vi "Main.vi"(8 "error in":errorcluster, 11 "Camera detection in":refnum<class "Camera detection.lvclass">) -> (0 "error out":errorcluster, 3 "Camera detection out":refnum<class "Camera detection.lvclass">)   [LabVIEW 2026, in "Camera detection.lvclass"]
doc: "The <b>Queued Message Handler</b> of the Worker that owns this VI."
uses:
  Camera detection.lvclass
  C:/Program Files/National Instruments/LabVIEW 2026/vi.lib/addons/_Workers/Library/Classes/Worker/Worker.lvclass
  Initialization Data.ctl
  Response Cases.ctl
  Camera detection.lvclass/Camera detection.ctl
  rql_Open Camera.ctl
  81cbe082-1300-4c77-b04d-38d83d7810f2.vi
  <vilib>/Utility/error.llb/Error Cluster From Error Code.vi
  <vilib>/ErrorRing/Error Ring.xnode
  <vilib>/addons/_Workers/Library/Classes/Message Queue/Message Queue.lvclass
  <vilib>/addons/_Workers/Debugger/Debug Client/Debug Client.lvlib
  <vilib>/Serenial/G Industrial Camera/g_industrial_cam/g_industrial_cam.lvlib
panel:
  out "élément":string
  in  "Open":bool
  in  "Caméra Identifiée":u16(ring) items=["Basler-acA640-120gm-22026460", "Basler-acA640-121gm-40611192"]
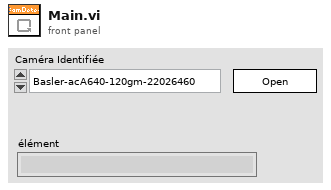
[diagram p1: front panel]
types:
  T1 = typedef "Camera detection.lvclass/Initialization Data.ctl" = cluster{"Response Cases":T2}
  T2 = typedef "Camera detection.lvclass/Response Cases.ctl" = cluster{"Placeholder - Can be deleted":string, "Non du VI":string, "Refnum Caméra ID":refnum<vi>}
  T3 = typedef "Camera detection.lvclass/rql_Open Camera.ctl" = cluster{"String":string, "Incr":i32}
  T4 = typedef "g_industrial_cam.lvlib/Device Enumeration.ctl" = cluster{"ID":string, "Protocol":string, "Vendor":string, "Model":string, "Serial":string, "Address":string}
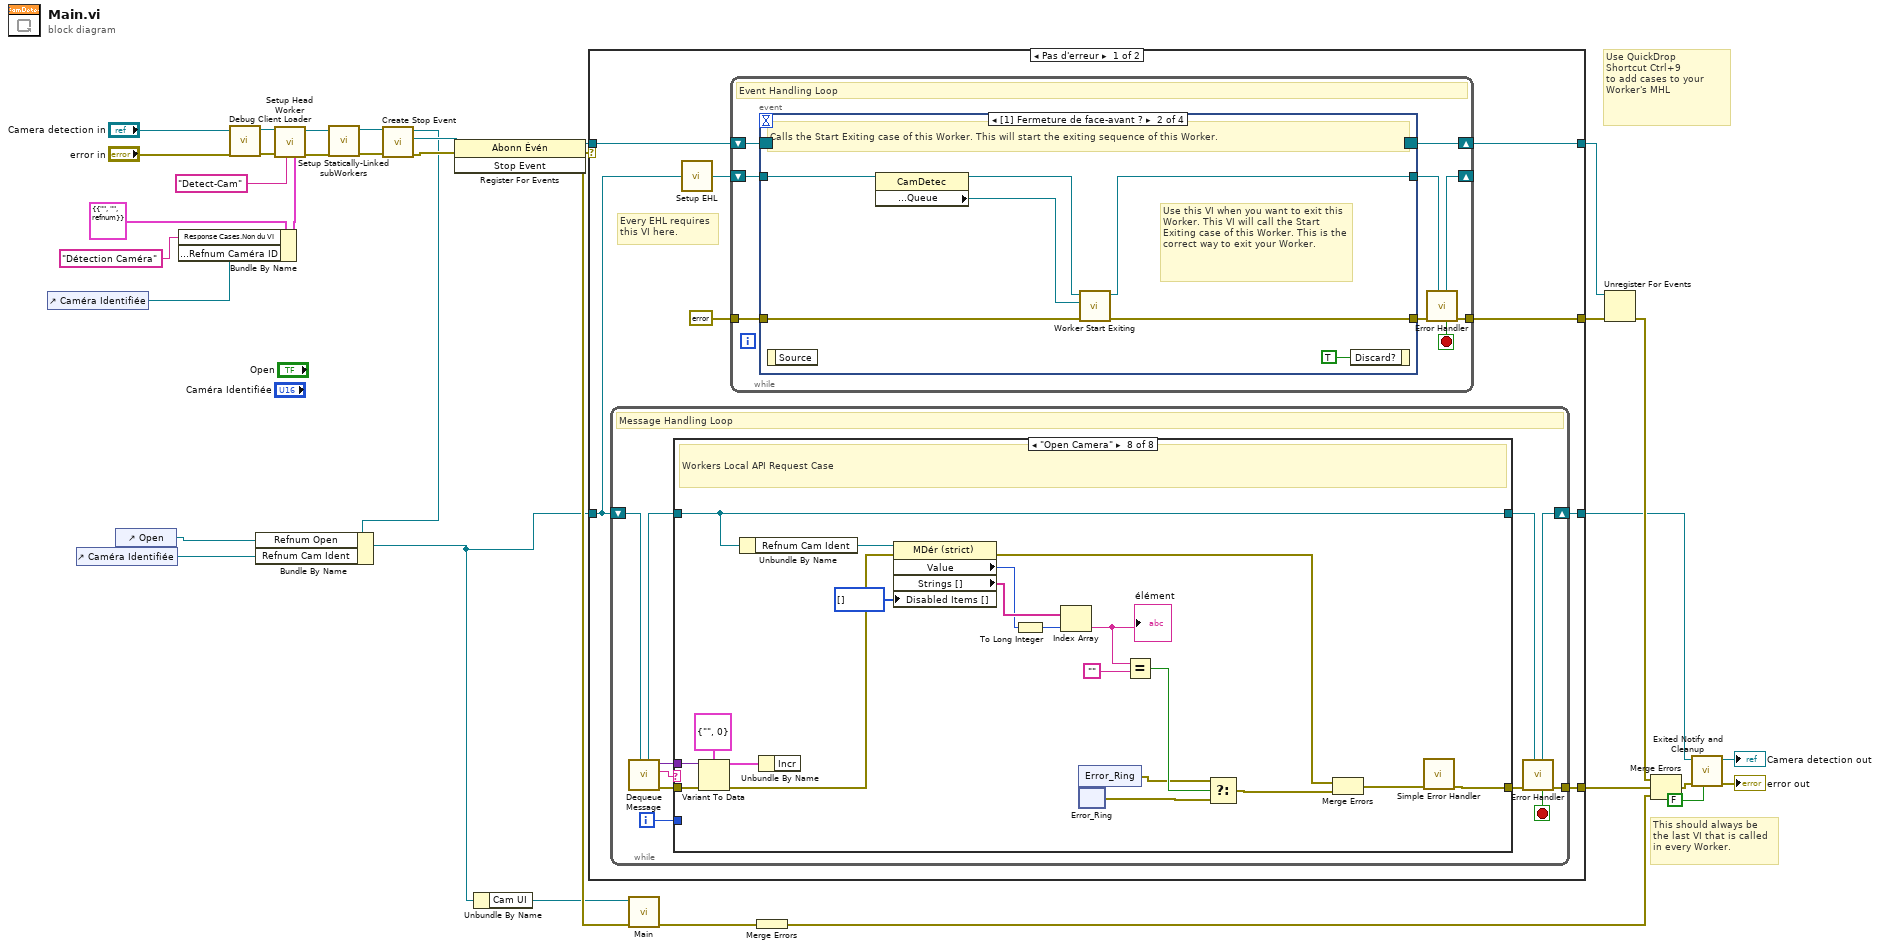
[diagram p0: block diagram]
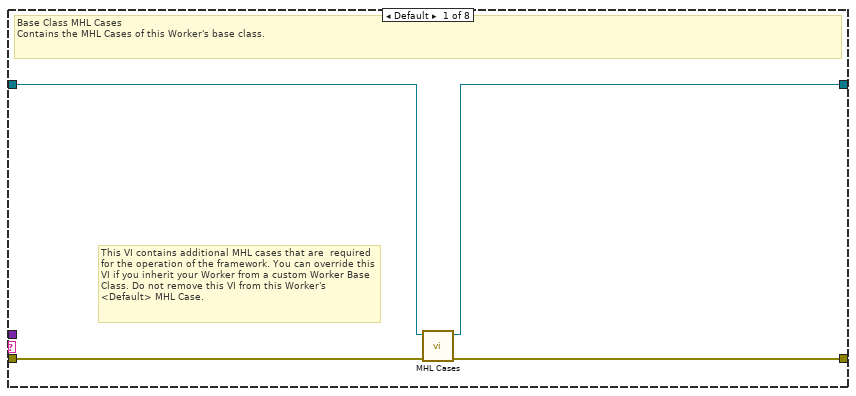
[diagram p2: hidden frame]
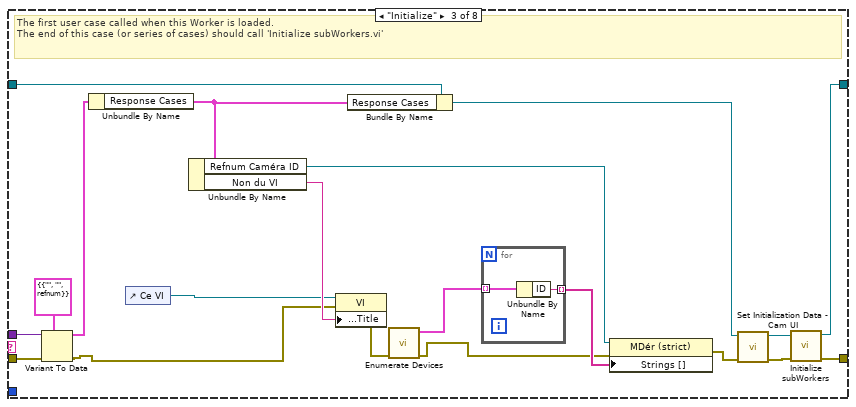
[diagram p4: hidden frame]
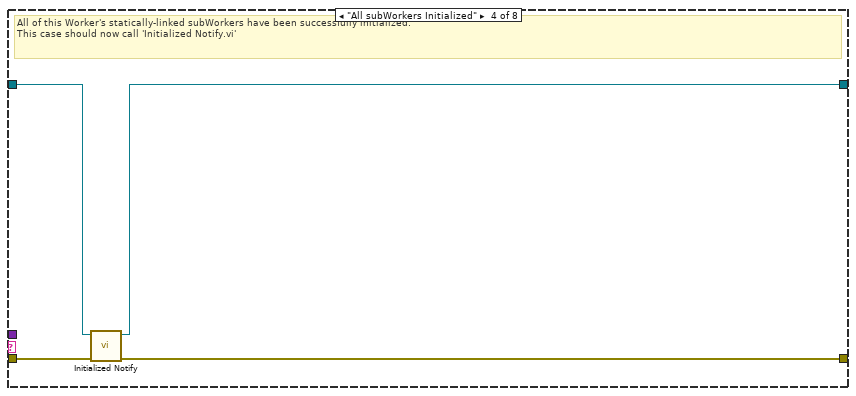
[diagram p5: hidden frame]
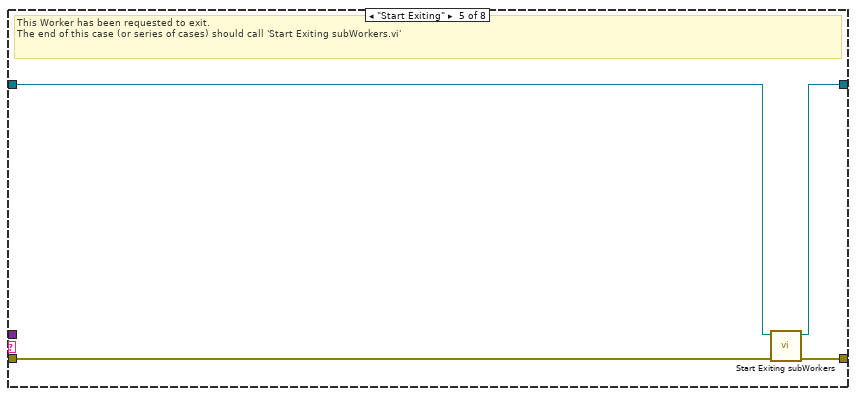
[diagram p6: hidden frame]
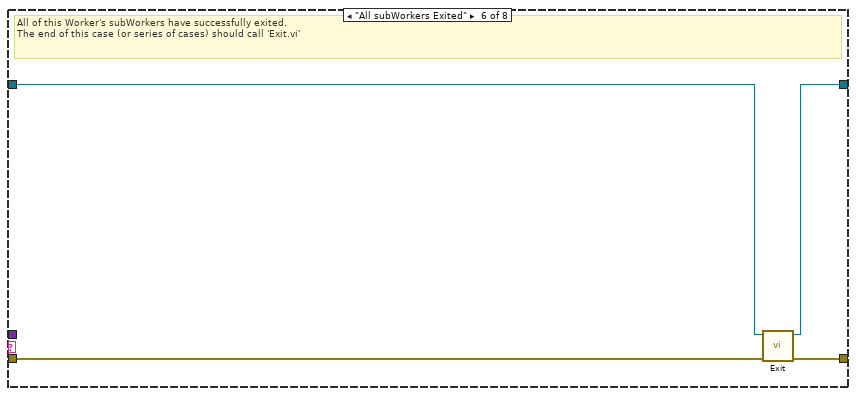
[diagram p7: hidden frame]
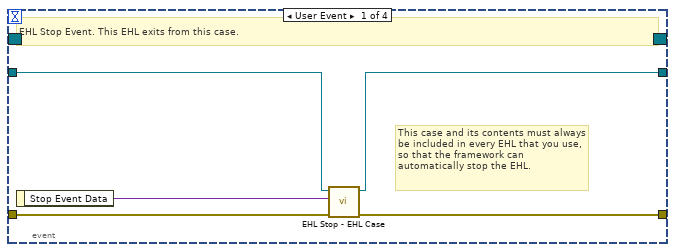
[diagram p9: hidden frame]
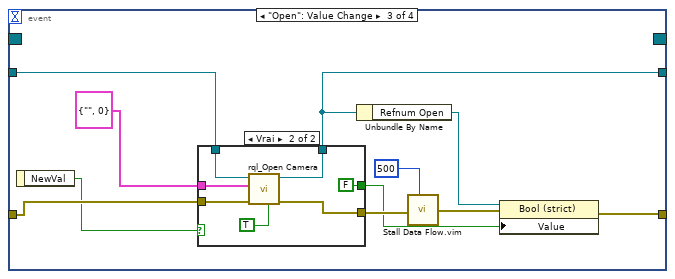
[diagram p10: hidden frame]
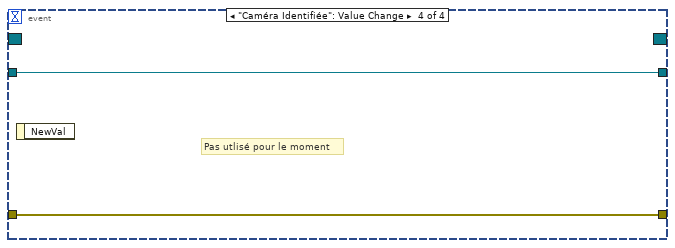
[diagram p12: hidden frame]
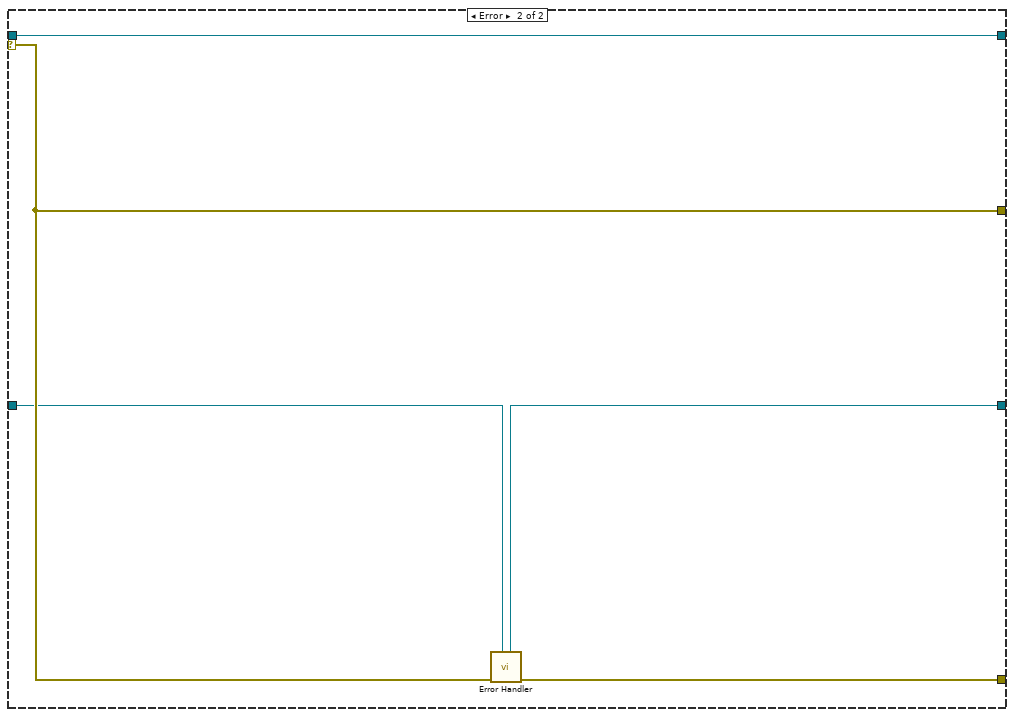
[diagram p13: hidden frame]
diagram:
  # "Use QuickDrop\nShortcut Ctrl+9\nto add cases to your\nWorker's MHL"
  # "This should always be the last VI that is called in every Worker."
  n1 = control-ref of="Caméra Identifiée"() -> (w13:refnum<vi>)
  n2 = control-ref of="Caméra Identifiée"() -> (w10:refnum<vi>)
  n3 = control-ref of="Open"() -> (w11:refnum<vi>)
  n4 = Bundle By Name ("Assembler par nom")(cluster=T1 {"Response Cases"={"Placeholder - Can be deleted"="", "Non du VI"="", "Refnum Caméra ID"=refnum}} ("Initialization Data"), "Response Cases.Non du VI"="Détection Caméra", "Response Cases.Refnum Caméra ID"=w13) -> (w16:T1)
  n5 = call <vilib>:"Debug Client Loader.vi"("error in (no error)"="error in", "Worker_"="Camera detection in") -> ("error out"=w19:errorcluster, "Worker_out"=w20:refnum<class "Camera detection.lvclass">)  [unwired: 8 in]
  n6 = call-dynamic "Setup Head Worker.vi"("Initalization Data"=w16, "Worker Alias"="Detect-Cam", "error in"=w19, "Worker_"=w20) -> ("error out"=w4:errorcluster, "Worker_out"=w3:refnum<class "Camera detection.lvclass">)  [unwired: 6 in]
  n7 = call "Setup Statically-Linked subWorkers.vi"("error in"=w4, "Camera detection in"=w3) -> ("error out"=w1:errorcluster, "Camera detection out"=w2:refnum<class "Camera detection.lvclass">)  [unwired: 8 in]
  n8 = call-dynamic "Create Stop Event.vi"("error in"=w1, "Worker"=w2) -> ("error out"=w28:errorcluster, "Stop Event"=w25:refnum<user-event>, "Worker out"=w22:refnum<class "Camera detection.lvclass">)  [unwired: 7 in]
  n9 = Bundle By Name ("Assembler par nom")(cluster=w22, "Refnum Open"=w11, "Refnum Cam Ident"=w10) -> (w12:refnum<class "Camera detection.lvclass">)
  n10 = register-events(error in=w28, w25) -> (reference out=w27:refnum<event-registration>, error out=w21:errorcluster)  [unwired: 1 in]
  n11 = Unbundle By Name(w12) -> ("Cam UI"=w7:refnum<class "Caméra UI.lvclass">)
  n12 = case shown="Pas d'erreur" w21 {
    tunnel: w12 -> [w36 w165]
    tunnel: [w34 w166] -> w26
    tunnel: w27 -> [w41 w167]
    tunnel: [w38 w168] -> w32
    tunnel: [w40 w167] -> w31
    tunnel: [w35 w164] -> w29
    selector: w21 -> [_ w168]
    frame No Error {
      # "Every EHL requires\nthis VI here."
      n13 = while {
        shift-right: [w50] -> w35
        shift-left: w36 -> [w52]
        tunnel: [w51] -> w34
        i -> [w43]
        stop <- w44 stop-if-true
        # "Message Handling Loop"
        n14 = call-dynamic "Dequeue Message.vi"("Worker"=w52) -> ("error out"=w49:errorcluster, "Case out"=w45:string, "Data out"=w42:variant, "Worker out"=w47:refnum<class "Camera detection.lvclass">)  [unwired: 6 in, 1 out]
        n15 = case "Worker MHL Case Structure (DO NOT CHANGE LABEL NAME)" shown="\"Open Camera\"" w45 {
          tunnel: w49 -> [w56 w57 w76 w82 w85 w92 w94 w114]
          tunnel: [w55 w57 w78 w81 w88 w91 w94 w98] -> w48
          tunnel: w47 -> [w54 w58 w75 w84 w86 w90 w93 w110]
          tunnel: [w53 w58 w77 w83 w87 w89 w93 w110] -> w46
          tunnel: w43 -> [_ _ _ _ _ _ _ _]
          tunnel: w42 -> [_ _ w74 _ _ _ _ w112]
          frame Default {
            # "This VI contains additional MHL cases that are  required for the operation of the framework. You can override this VI if you inherit your Worker from a custom Worker Base Class. Do not remove this VI from this Worker's <Default> MHL Case."
            # "Base Class MHL Cases\nContains the MHL Cases of this Worker's base class."
            n16 = call-dynamic "MHL Cases.vi"("error in"=w56, "Worker in"=w54) -> ("error out"=w55:errorcluster, "Worker out"=w53:refnum<class "Camera detection.lvclass">)  [unwired: 8 in]
          }
          frame "------------ FRAMEWORK CASES -----------" {
            # "Start of Workers Framework Cases"
          }
          frame "Initialize" {
            # "The first user case called when this Worker is loaded.\nThe end of this case (or series of cases) should call 'Initialize subWorkers.vi'"
            n17 = Variant To Data(error in=w76, type=T1 {"Response Cases"={"Placeholder - Can be deleted"="", "Non du VI"="", "Refnum Caméra ID"=refnum}} ("Initialization Data"), Variant=w74) -> (data=w73:T1, error out=w67:errorcluster)
            n18 = Unbundle By Name(w73) -> ("Response Cases"=w68:T2)
            n19 = control-ref of="Ce VI"() -> (w63:refnum<vi>)
            n20 = Unbundle By Name(w68) -> ("Refnum Caméra ID"=w65:refnum<vi>, "Non du VI"=w71:string)
            n21 = property class="VI"(reference=w63, error in=w67, "Front Panel.Title"=w71) -> (error out=w70:errorcluster)  [unwired: 1 out]
            n22 = Bundle By Name ("Assembler par nom")(cluster=w75, "Response Cases"=w68) -> (w59:refnum<class "Camera detection.lvclass">)
            n23 = call <vilib>:"Enumerate Devices.vi"("error in (no error)"=w70) -> ("error out"=w62:errorcluster, "Devices"=w69:T4[])  [unwired: 9 in]
            n24 = for {
              tunnel: w69 -> [w80] mode=indexing
              tunnel: [w79] -> w64 mode=indexing
              n25 = Unbundle By Name(w80) -> ("ID"=w79:string)
            }
            n26 = property class="MDér (strict)"(reference=w65, error in=w62, "Strings []"=w64) -> (error out=w66:errorcluster)  [unwired: 1 out]
            n27 = call "Set Initialization Data - Cam UI.vi"("error in"=w66, "Camera detection in"=w59) -> ("error out"=w61:errorcluster, "Camera detection out"=w60:refnum<class "Camera detection.lvclass">)  [unwired: 8 in]
            n28 = call-dynamic "Initialize subWorkers.vi"("error in"=w61, "Worker"=w60) -> ("error out"=w78:errorcluster, "dup Worker out"=w77:refnum<class "Camera detection.lvclass">)  [unwired: 8 in]
          }
          frame "All subWorkers Initialized" {
            # "All of this Worker's statically-linked subWorkers have been successfully initialized.\nThis case should now call 'Initialized Notify.vi'"
            n29 = call-dynamic "Initialized Notify.vi"("error in"=w82, "Worker"=w84) -> ("error out"=w81:errorcluster, "dup Worker out"=w83:refnum<class "Camera detection.lvclass">)  [unwired: 8 in]
          }
          frame "Start Exiting" {
            # "This Worker has been requested to exit. \nThe end of this case (or series of cases) should call 'Start Exiting subWorkers.vi'"
            n30 = call-dynamic "Start Exiting subWorkers.vi"("error_in"=w85, "Worker"=w86) -> ("error out"=w88:errorcluster, "dup Worker out"=w87:refnum<class "Camera detection.lvclass">)  [unwired: 8 in]
          }
          frame "All subWorkers Exited" {
            # "All of this Worker's subWorkers have successfully exited. \nThe end of this case (or series of cases) should call 'Exit.vi'"
            n31 = call-dynamic "Exit.vi"("error_in"=w92, "Worker"=w90) -> ("error out"=w91:errorcluster, "dup Worker out"=w89:refnum<class "Camera detection.lvclass">)  [unwired: 8 in]
          }
          frame "------------- LOCAL API CASES -------------" {
            # "Start of Workers Local API Cases"
          }
          frame "Open Camera" {
            # "Workers Local API Request Case"
            n32 = Variant To Data(error in=w114, type=T3 {"String"="", "Incr"=0} ("Data"), Variant=w112) -> (data=w111:T3, error out=w108:errorcluster)
            n33 = Unbundle By Name(w110) -> ("Refnum Cam Ident"=w109:refnum<vi>)
            n34 = Unbundle By Name(w111) -> ()  [unwired: 1 out]
            n35 = property class="MDér (strict)"(reference=w109, error in=w108, "Disabled Items []"=i32[] [] ("Éléments désactivés []")) -> (error out=w107:errorcluster, "Value"=w105:u16, "Strings []"=w106:string[])  [unwired: 1 out]
            n36 = To Long Integer(number=w105) -> (32bit integer=w96:i32)
            n37 = Index Array(array=w106, index=w96) -> (element=w95:string)
            "élément" <- w95
            n38 = xnode ("Error_Ring")() -> ("sortie d'erreur"=w102:errorcluster)
            n39 = xnode ("Error_Ring")() -> ("sortie d'erreur"=w101:errorcluster)
            n40 = Equal?(x=w95, y="") -> (x = y?=w103:bool)
            n41 = Select(t=w102, s=w103, f=w101) -> (s? t:f=w100:errorcluster)
            n42 = Merge Errors ("Fusionner les erreurs")(w107, w100) -> (w99:errorcluster)
            n43 = call <vilib>:"Simple Error Handler.vi"("error in (no error)"=w99) -> ("error out"=w98:errorcluster)  [unwired: 4 in, 4 out]
          }
        }
        n44 = call-dynamic "Error Handler.vi"("Worker"=w46, "error_in"=w48) -> ("error out"=w51:errorcluster, "Stop Loop"=w44:bool, "Worker out"=w50:refnum<class "Camera detection.lvclass">)  [unwired: 7 in]
      }
      n45 = call-dynamic "Setup EHL.vi"("Worker"=w36) -> ("Worker out"=w37:refnum<class "Camera detection.lvclass">)  [unwired: 14 in]
      n46 = while "Event Handling Loop" {
        shift-right: [w129] -> w40
        shift-left: w41 -> [w128]
        tunnel: [w124] -> w38
        tunnel: errorcluster {"status"=FALSE, "code"=0, "source"=""} ("error constant") -> [w126]
        shift-right: [w122] -> _
        shift-left: w37 -> [w127]
        stop <- w121 stop-if-true
        # "Event Handling Loop"
        n47 = event shown="[1] Fermeture de face-avant ?" {
          selector: w128 -> [_ _ _ _]
          dyn-events: [_ _ _ _] -> w129
          timeout: _ -> [_ _ _ _]
          tunnel: [w133 w140 w148 w163] -> w125
          tunnel: w126 -> [w134 w139 w152 w163]
          tunnel: w127 -> [w132 w138 w151 w162]
          tunnel: [w131 w137 w147 w162] -> w123
          event User Event {
            # "This case and its contents must always be included in every EHL that you use, so that the framework can automatically stop the EHL."
            # "EHL Stop Event. This EHL exits from this case."
            n48 = event-data() -> ("Stop Event Data"=w130:variant)  [unwired: 1 in]
            n49 = call-dynamic "EHL Stop - EHL Case.vi"("error in"=w134, "Stop Event Data"=w130, "Worker"=w132) -> ("error out"=w133:errorcluster, "Worker out"=w131:refnum<class "Camera detection.lvclass">)  [unwired: 7 in]
          }
          event Panel Close? {
            # "Use this VI when you want to exit this Worker. This VI will call the Start Exiting case of this Worker. This is the correct way to exit your Worker."
            # "Calls the Start Exiting case of this Worker. This will start the exiting sequence of this Worker."
            n50 = event-data() -> ()  [unwired: 1 in, 1 out]
            n51 = property class="CamDetec"(reference=w138) -> (reference out=w136:refnum<class "Camera detection.lvclass">, "Accessors:Read:Public API:Queue"=w135:refnum<class "Message Queue.lvclass">)  [unwired: 1 in, 1 out]
            n52 = call-dynamic "Worker Start Exiting.vi"("error_in"=w139, "Message Queue"=w135, "Worker"=w136) -> ("error out"=w140:errorcluster, "dup Worker out"=w137:refnum<class "Camera detection.lvclass">)  [unwired: 7 in]
            n53 = event-data ("Nœud de filtre d'événements")("Discard?"=TRUE) -> ()  [unwired: 1 in, 1 out]
          }
          event "Open": Value Change {
            n54 = event-data() -> ("NewVal"=w149:bool)  [unwired: 1 in]
            n55 = case shown="Vrai" w149 {
              tunnel: w152 -> [w154 w161]
              tunnel: [w154 w160] -> w145
              tunnel: w151 -> [w153 w159]
              tunnel: T3 {"String"="", "Incr"=0} ("Data in") -> [_ w158]
              tunnel: [w153 w157] -> w147
              tunnel: [_ FALSE ("Show in Debugger?")] -> w143
              frame False {
              }
              frame True {
                n56 = call "rql_Open Camera.vi"("Show in Debugger?"=TRUE, "error in"=w161, "Data in"=w158, "Camera detection in"=w159) -> ("error out"=w160:errorcluster, "dup Camera detection out"=w157:refnum<class "Camera detection.lvclass">)  [unwired: 6 in]
              }
            }
            n57 = Unbundle By Name(w147) -> ("Refnum Open"=w146:refnum<vi>)
            n58 = call "Stall Data Flow.vim"("value in"=w145, "milliseconds to wait"=u32 500) -> ("value out"=w144:errorcluster)  [unwired: 1 out]
            n59 = property class="Bool (strict)"(reference=w146, error in=w144, "Value"=w143) -> (error out=w148:errorcluster)  [unwired: 1 out]
          }
          event "Caméra Identifiée": Value Change {
            # "Pas utlisé pour le moment"
            n60 = event-data() -> ()  [unwired: 1 in, 1 out]
          }
        }
        n61 = call-dynamic "Error Handler.vi"("Worker"=w123, "error_in"=w125) -> ("error out"=w124:errorcluster, "Stop Loop"=w121:bool, "Worker out"=w122:refnum<class "Camera detection.lvclass">)  [unwired: 7 in]
      }
    }
    frame Error {
      n62 = call-dynamic "Error Handler.vi"("Worker"=w165, "error_in"=w168) -> ("error out"=w166:errorcluster, "Worker out"=w164:refnum<class "Camera detection.lvclass">)  [unwired: 7 in, 1 out]
    }
  }
  n63 = call-dynamic "Main.vi"("error in"=w21, "Caméra UI in"=w7) -> ("error out"=w9:errorcluster)  [unwired: 8 in, 1 out]
  n64 = Merge Errors(w9) -> (w8:errorcluster)
  n65 = Unregister For Events(event registration refnum=w31, error in=w32) -> (error out=w33:errorcluster)
  n66 = Merge Errors ("Fusionner les erreurs")(w33, w26, w8) -> (w30:errorcluster)
  n67 = call-dynamic "Exited Notify and Cleanup.vi"("Close FP on Exit? (T)"=FALSE, "error_in"=w30, "Worker"=w29) -> ("error out"=→"error out":errorcluster, "dup Worker out"=→"Camera detection out":refnum<class "Camera detection.lvclass">)  [unwired: 7 in]
